vi "Read_raw_inst_setup.vi"(0 "Setup file":path) -> (5 "Board type":T4=enum."NB-MIO-16H", 6 "Local ADAM Channels":string[](array[string]), 8 "Setup string":string, 10 "Ch & spans choices":T5(array[cluster]) {"D" format="%.2f"; "Ch No" min=0; "low limit (-10V)" min=-10 max=10 format="%.2f"; "high limit (10V)" min=-10 max=10 format="%.2f"}, 13 "PWA Data":T1, 14 "Number of Analogue instruments":i32=1, 16 "LDA data":enum16{"No LDA data", "Take LDA data"}(ring)=enum."Take LDA data", 17 "LDA set up":T3={"dimensions"=enum."2D", "Arrival spacing"=FALSE, "Transit time"=FALSE}, 19 "Synchronise Analogue channels with LDA":bool)   [LabVIEW 2010]
uses:
  Controls/Inst_type.ctl
  Controls/Board_Types.ctl
  Controls/PWA_Data.ctl
  Controls/Post_Process.ctl
  Controls/Trigger_Mode.ctl
  Controls/Tunnel_Coordinates.ctl
  Globals/Meas_global.vi
  Globals/LDA_meas_global_1.vi
  Globals/LDA_meas_global_2.vi
  Globals/Trav_pos_global.vi
panel:
  in  "Inst type":T2
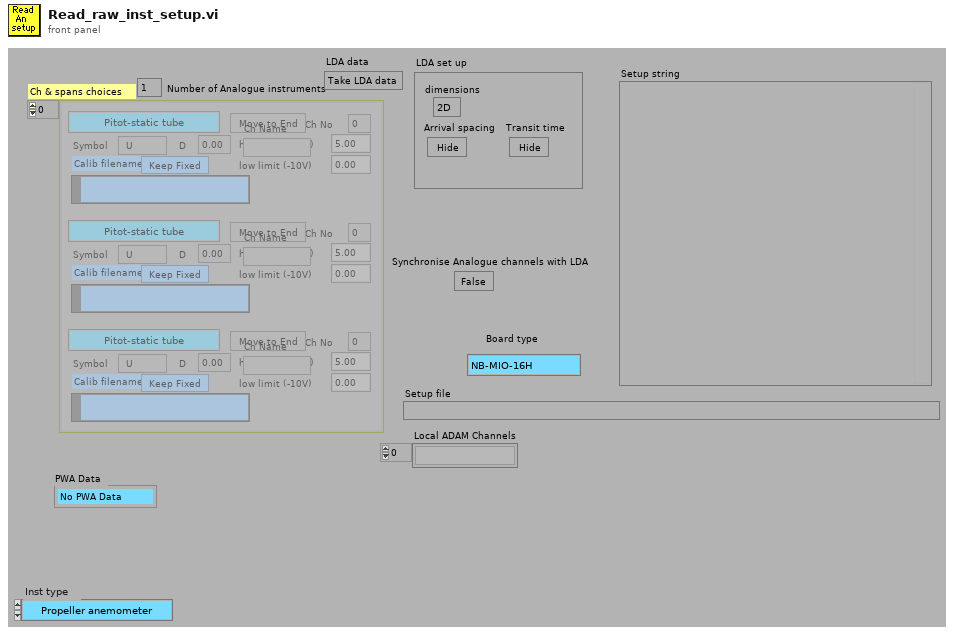
[diagram p1: front panel]
types:
  T1 = typedef "PWA_Data.ctl" = enum16{"No PWA Data", "One Ch PWA"}
  T2 = typedef "Inst_type.ctl" = enum16{"Propeller anemometer", "Raw voltage", "Pressure Transducer", "Pitot-static tube", "Preston tube", "Hot wire", "Cross wire 1", "Cross wire 2", "Generic Linear", "Generic Polynomial", "Generic BackPoly", "Fast FID", "Thermocouple", "Cold wire", "Pulsed Wire", "LDA Vel", "LDA Tran time", "LDA Arr time"}
  T3 = cluster{"dimensions":enum16{"1D", "2D"}, "Arrival spacing":bool, "Transit time":bool}
  T4 = typedef "Board_Types.ctl" = enum16{"Simulate", "NB-MIO-16H", "PCI-MIO-16E", "6000E Series", "USB-92xx", "ADC488", "Lab-NB", "NB-DIO-24", "NI-DAQmx", "Local ADAM", "Server Channels"}
  T5 = cluster{"high limit (10V)":sgl, "low limit (-10V)":sgl, "Ch No":i16, "Calib filename":path, "Inst type":T2, "Symbol":string, "Move channel":bool, "Use Latest":bool, "D":dbl, "Ch Name":string}[]
  T6 = typedef "Post_Process.ctl" = enum16{"Take New Data", "Post Process Raw Data File"}
  T7 = typedef "Trigger_Mode.ctl" = enum16{"Free Running", "Start on Trigger", "Trigger Every Block", "Trigger Every Sample"}
  T8 = typedef "Tunnel_Coordinates.ctl" = enum16{"Work in Tunnel Coordinates", "Work in Model Coordinates"}
  T9 = cluster{"high limit (10V)":sgl, "low limit (-10V)":sgl, "Ch No":i16, "Calib filename":path, "Inst type":T2, "Symbol":string, "Move channel":bool, "Use Latest":bool, "D":dbl, "Ch Name":string}
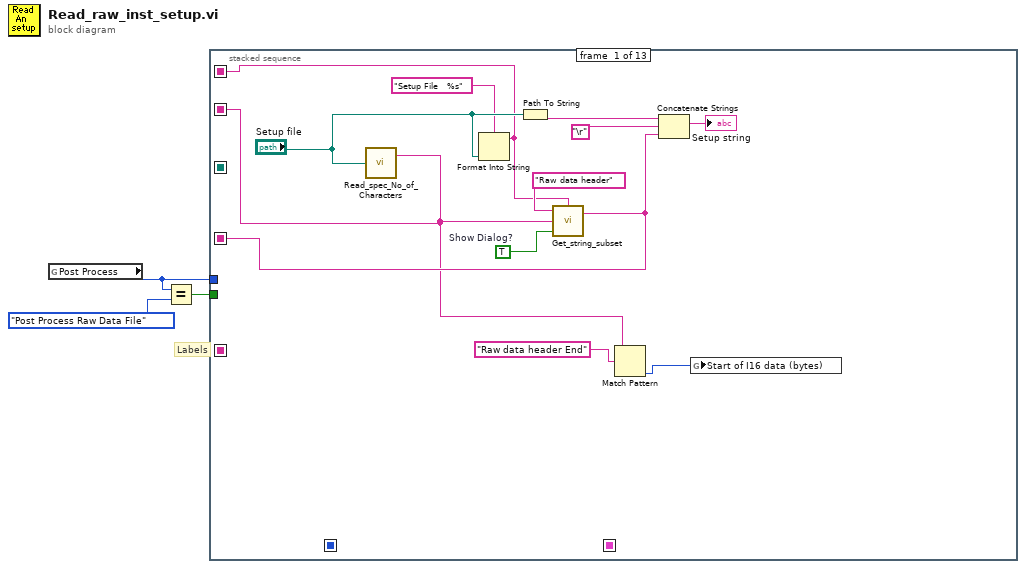
[diagram p0: block diagram]
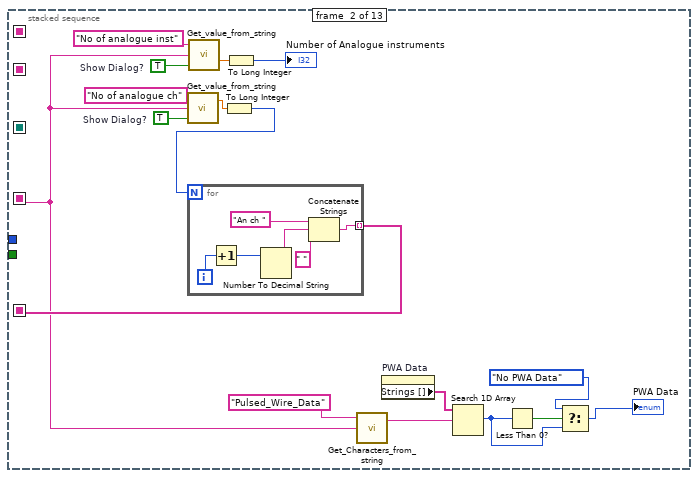
[diagram p2: hidden frame]
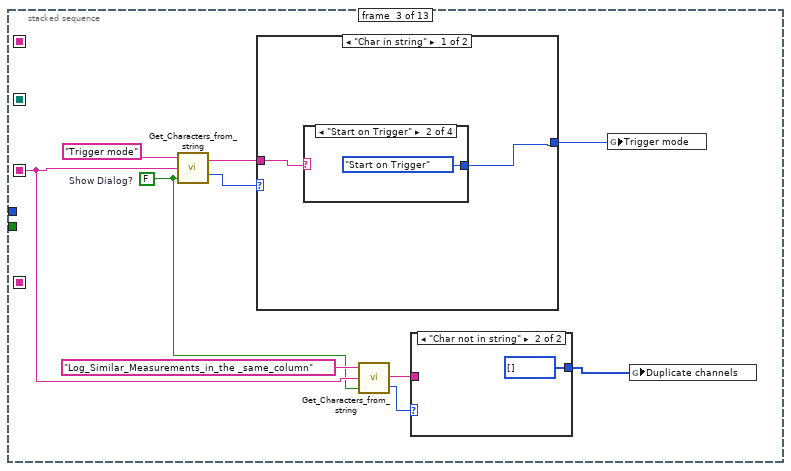
[diagram p3: hidden frame]
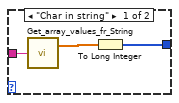
[diagram p4: hidden frame]
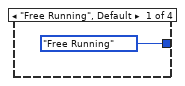
[diagram p5: hidden frame]
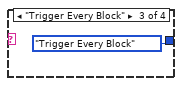
[diagram p6: hidden frame]
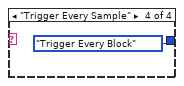
[diagram p7: hidden frame]
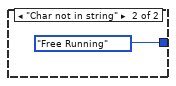
[diagram p8: hidden frame]
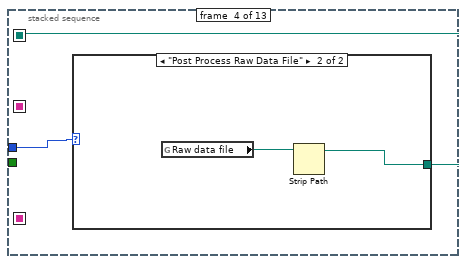
[diagram p9: hidden frame]
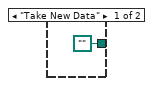
[diagram p10: hidden frame]
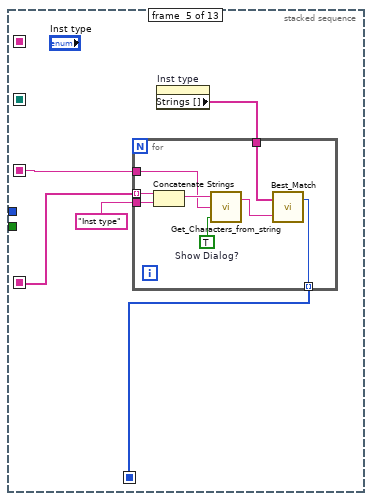
[diagram p11: hidden frame]
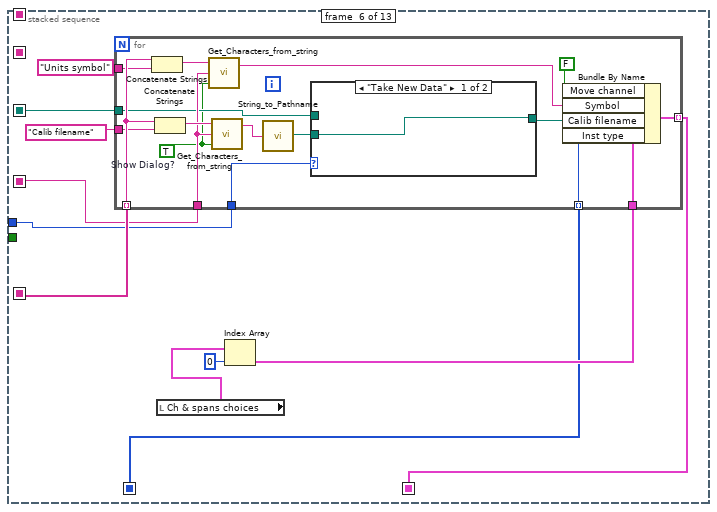
[diagram p12: hidden frame]
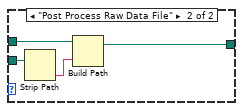
[diagram p13: hidden frame]
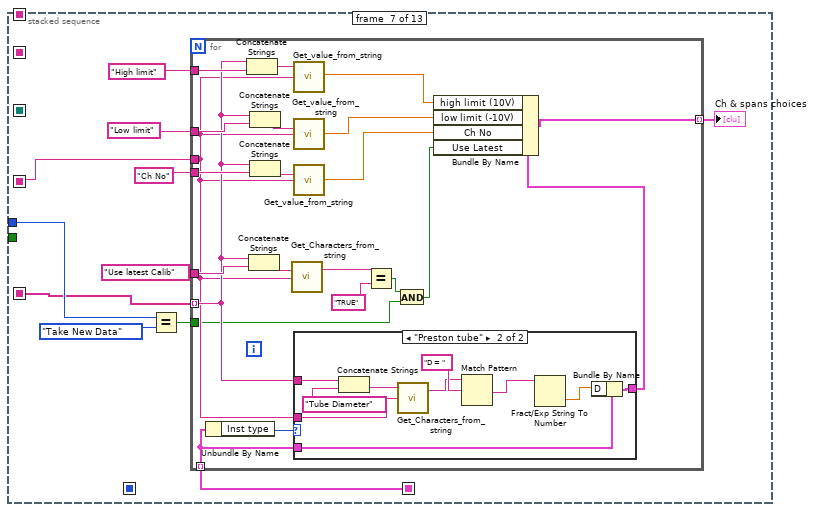
[diagram p14: hidden frame]
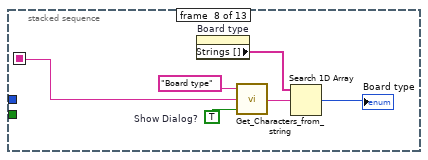
[diagram p16: hidden frame]
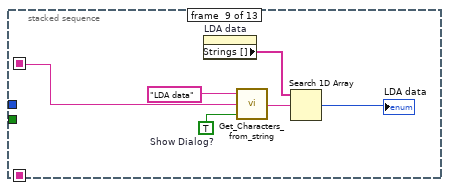
[diagram p17: hidden frame]
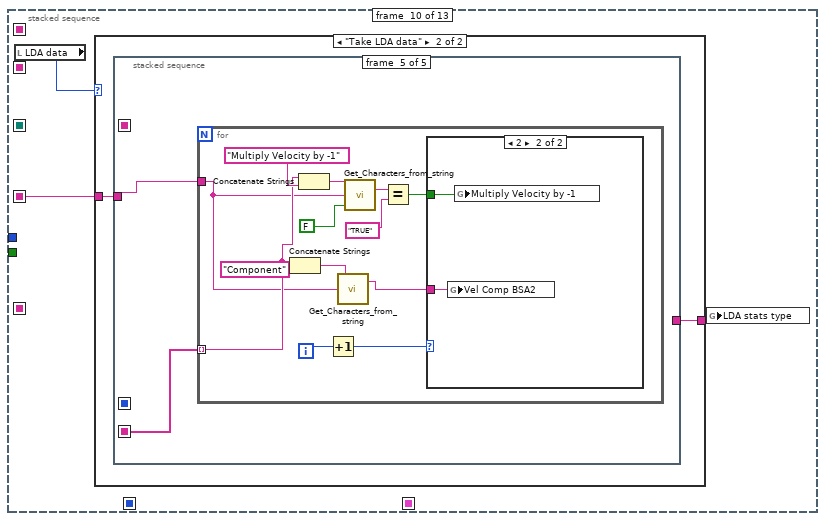
[diagram p18: hidden frame]
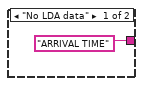
[diagram p19: hidden frame]
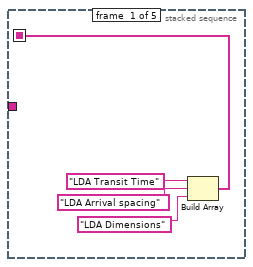
[diagram p20: hidden frame]
diagram:
  # "Labels"
  n1 = global read "Meas_global.vi" "Post Process"() -> (w1:T6)
  n2 = Equal?(x=w1, y=Post_Process."Post Process Raw Data File" ("Post Process")) -> (x = y?=w3:bool)
  n3 = stacked-sequence {
    seq-local: [w13 _ _ _ _ _ _ _ _ _ _ _ _] -> [_ w23 w43 _ w69 w79 w121 w159 w165 w169 w251 w278 w291]
    seq-local: [_ w30 _ _ _ _ _ _ _ _ _ _ _] -> [_ _ _ _ w68 w88 w112 _ _ _ _ _ _]
    seq-local: [_ _ _ _ w65 _ _ _ _ _ _ _ _] -> [_ _ _ _ _ w82 _ _ _ _ _ _ _]
    seq-local: [_ _ _ _ _ w81 _ _ _ _ _ _ _] -> [_ _ _ _ _ _ w120 _ _ _ _ _ _]
    seq-local: [_ _ _ w61 _ _ _ _ _ _ _ _ _] -> [_ _ _ _ _ w80 _ _ _ _ _ _ _]
    seq-local: [w8 _ _ _ _ _ _ _ _ _ _ _ _] -> [_ _ _ _ _ _ _ _ _ _ _ _ w290]
    seq-local: [w4 _ _ _ _ _ _ _ _ _ _ _ _] -> [_ _ _ _ _ _ _ _ _ _ _ w274 _]
    tunnel: w3 -> [_ _ _ _ _ _ _ _ _ _ _ _ w292]
    tunnel: w1 -> [_ _ _ w60 _ w78 w113 _ _ _ _ w275 _]
    frame #0 {
      w10 = TRUE  # Show Dialog?
      n4 = call "Read_spec_No_of_Characters.vi"("Filename"="Setup file") -> ("character string"=w8:string)  [unwired: 1 out]
      n5 = Format Into String(format string="Setup File   %s", "Setup file") -> (resulting string=w4:string)  [unwired: 2 in, 1 out]
      n6 = Path To String(path="Setup file") -> (string=w11:string)
      n7 = call "Get_string_subset.vi"("String Name"=w4, "Show Dialog?"=w10, "String to split"=w8, "File Label"="Raw data header") -> ("Output string"=w13:string)  [unwired: 1 out]
      n8 = Match Pattern(string=w8, regular expression="Raw data header End") -> (offset past match=w7:i32)  [unwired: 4 out]
      n9 = Concatenate Strings(w11, "\r", w13) -> (→"Setup string":string)
      n10 = global write "Meas_global.vi" "Start of I16 data (bytes)"(w7) -> ()
    }
    frame #1 {
      w24 = TRUE  # Show Dialog?
      w25 = TRUE  # Show Dialog?
      n11 = call "Get_value_from_string.vi"("Show Dialog?"=w25, "Input string"=w23, "Variable name"="No of analogue ch") -> ("Value"=w31:dbl)  [unwired: 1 out]
      n12 = call "Get_value_from_string.vi"("Show Dialog?"=w24, "Input string"=w23, "Variable name"="No of analogue inst") -> ("Value"=w28:dbl)  [unwired: 1 out]
      n13 = To Long Integer(number=w31) -> (32bit integer=w26:i32)
      n14 = for {
        N: w26 -> [_]
        tunnel: [w34] -> w30 mode=indexing
        i -> [w36]
        n15 = Increment(x=w36) -> (x+1=w35:i32)
        n16 = Number To Decimal String(number=w35) -> (decimal integer string=w38:string)  [unwired: 1 out]
        n17 = Concatenate Strings("An ch ", w38, " ") -> (w34:string)
      }
      n18 = To Long Integer(number=w28) -> (32bit integer=→"Number of Analogue instruments":i32)
      n19 = call "Get_Characters_from_string.vi"("Input string"=w23, "Variable name"="Pulsed_Wire_Data") -> ("Value"=w20:string)  [unwired: 1 in, 1 out]
      n20 = property on="PWA Data" class="Enum (strict)"() -> ("Strings []"=w21:string[])  [unwired: 2 in, 2 out]
      n21 = Search 1D Array(1D array=w21, element=w20) -> (index of element=w17:i32)  [unwired: 1 out]
      n22 = Less Than 0?(x=w17) -> (x < 0?=w19:bool)
      n23 = Select(t=PWA_Data."No PWA Data" ("PWA Data"), s=w19, f=w17) -> (s? t:f=→"PWA Data":i32)
    }
    frame #2 {
      w42 = FALSE  # Show Dialog?
      n24 = call "Get_Characters_from_string.vi"("Show Dialog?"=w42, "Input string"=w43, "Variable name"="Trigger mode") -> ("Status"=w47:enum16{"Char in string", "Char not in string"}, "Value"=w46:string)
      n25 = case shown="\"Char in string\"" w47 {
        tunnel: [w53 Trigger_Mode."Free Running" ("Trigger mode")] -> w45
        tunnel: w46 -> [w54 _]
        frame "Char in string" {
          n26 = case shown="\"Start on Trigger\"" w54 {
            tunnel: [Trigger_Mode."Free Running" ("Trigger mode") Trigger_Mode."Start on Trigger" ("Trigger mode") Trigger_Mode."Trigger Every Block" ("Trigger mode") Trigger_Mode."Trigger Every Block" ("Trigger mode")] -> w53
            frame "Free Running", Default {
            }
            frame "Start on Trigger" {
            }
            frame "Trigger Every Block" {
            }
            frame "Trigger Every Sample" {
            }
          }
        }
        frame "Char not in string" {
        }
      }
      n27 = call "Get_Characters_from_string.vi"("Show Dialog?"=w42, "Input string"=w43, "Variable name"="Log_Similar_Measurements_in_the _same_column") -> ("Status"=w39:enum16{"Char in string", "Char not in string"}, "Value"=w41:string)
      n28 = case shown="\"Char not in string\"" w39 {
        tunnel: w41 -> [w51 _]
        tunnel: [w49 i32[] []] -> w40
        frame "Char in string" {
          n29 = call "Get_array_values_fr_String.vi"("String Value"=w51) -> ("Numeric Array"=w50:dbl[])  [unwired: 1 out]
          n30 = To Long Integer(number=w50) -> (32bit integer=w49:i32[])
        }
        frame "Char not in string" {
        }
      }
      n31 = global write "Meas_global.vi" "Trigger mode"(w45) -> ()
      n32 = global write "Meas_global.vi" "Duplicate channels"(w40) -> ()
    }
    frame #3 {
      n33 = case shown="\"Post Process Raw Data File\"" w60 {
        tunnel: [path "" ("stripped path") w63] -> w61
        frame "Take New Data" {
        }
        frame "Post Process Raw Data File" {
          n34 = global read "Meas_global.vi" "Raw data file"() -> (w64:path)
          n35 = Strip Path(path=w64) -> (stripped path=w63:path)  [unwired: 1 out]
        }
      }
    }
    frame #4 {
      n36 = property on="Inst type" class="Enum (strict)"() -> ("Strings []"=w66:string[])  [unwired: 2 in, 2 out]
      n37 = for {
        tunnel: w69 -> [w76]
        tunnel: w66 -> [w72]
        tunnel: w68 -> [w75] mode=indexing
        tunnel: "Inst type" -> [w74]
        tunnel: [w70] -> w65 mode=indexing
        w73 = TRUE  # Show Dialog?
        n38 = Concatenate Strings(w75, w74) -> (w77:string)
        n39 = call "Get_Characters_from_string.vi"("Show Dialog?"=w73, "Input string"=w76, "Variable name"=w77) -> ("Value"=w71:string)  [unwired: 1 out]
        n40 = call "Best_Match.vi"("Input String"=w71, "String Options"=w72) -> ("index of element"=w70:i32)  [unwired: 1 out]
      }
    }
    frame #5 {
      n41 = local read "Ch & spans choices"() -> (w84:T5)
      n42 = Index Array(array=w84, index=0) -> (element=w83:T9)
      n43 = for {
        tunnel: w88 -> [w103] mode=indexing
        tunnel: "Calib filename" -> [w102]
        tunnel: "Units symbol" -> [w101]
        tunnel: w83 -> [w100]
        tunnel: w82 -> [w98] mode=indexing
        tunnel: [w97] -> w81 mode=indexing
        tunnel: w79 -> [w96]
        tunnel: w78 -> [w95]
        tunnel: w80 -> [w94]
        w91 = TRUE  # Show Dialog?
        n44 = Concatenate Strings(w103, w101) -> (w105:string)
        n45 = Concatenate Strings(w103, w102) -> (w104:string)
        n46 = call "Get_Characters_from_string.vi"("Show Dialog?"=w91, "Input string"=w96, "Variable name"=w105) -> ("Value"=w99:string)  [unwired: 1 out]
        n47 = call "Get_Characters_from_string.vi"("Show Dialog?"=w91, "Input string"=w96, "Variable name"=w104) -> ("Value"=w90:string)  [unwired: 1 out]
        n48 = call "String_to_Pathname.vi"("Input String"=w90) -> ("path"=w89:path)
        n49 = case shown="\"Take New Data\"" w95 {
          tunnel: w89 -> [w106 w110]
          tunnel: w94 -> [_ w107]
          tunnel: [w106 w108] -> w93
          frame "Take New Data" {
          }
          frame "Post Process Raw Data File" {
            n50 = Strip Path(path=w110) -> (name=w109:string)  [unwired: 1 out]
            n51 = Build Path(base path=w107, name or relative path=w109) -> (appended path=w108:path)
          }
        }
        n52 = Bundle By Name(cluster=w100, "Move channel"=FALSE, "Symbol"=w99, "Calib filename"=w93, "Inst type"=w98) -> (w97:T9)
      }
    }
    frame #6 {
      n53 = Equal?(x=w113, y=Post_Process."Take New Data" ("Post Process")) -> (x = y?=w111:bool)
      n54 = for {
        tunnel: "Low limit" -> [w143]
        tunnel: "High limit" -> [w142]
        tunnel: w120 -> [w124] mode=indexing
        tunnel: [w134] -> w119 mode=indexing
        tunnel: w121 -> [w126]
        tunnel: "Ch No" -> [w138]
        tunnel: "Use latest Calib" -> [w132]
        tunnel: w112 -> [w127] mode=indexing
        tunnel: w111 -> [w125]
        n55 = Unbundle By Name(w124) -> ("Inst type"=w128:T2)
        n56 = Concatenate Strings(w127, w142) -> (w141:string)
        n57 = Concatenate Strings(w127, w132) -> (w133:string)
        n58 = Concatenate Strings(w127, w143) -> (w140:string)
        n59 = Concatenate Strings(w127, w138) -> (w139:string)
        n60 = call "Get_Characters_from_string.vi"("Input string"=w126, "Variable name"=w133) -> ("Value"=w131:string)  [unwired: 1 in, 1 out]
        n61 = call "Get_value_from_string.vi"("Input string"=w126, "Variable name"=w141) -> ("Value"=w137:dbl)  [unwired: 1 in, 1 out]
        n62 = call "Get_value_from_string.vi"("Input string"=w126, "Variable name"=w140) -> ("Value"=w136:dbl)  [unwired: 1 in, 1 out]
        n63 = call "Get_value_from_string.vi"("Input string"=w126, "Variable name"=w139) -> ("Value"=w135:dbl)  [unwired: 1 in, 1 out]
        n64 = case shown="\"Preston tube\"" w128 {
          tunnel: w127 -> [_ w154]
          tunnel: w126 -> [_ w149]
          tunnel: w124 -> [w144 w152]
          tunnel: [w144 w151] -> w123
          frame "Propeller anemometer", Default {
          }
          frame "Preston tube" {
            n65 = Concatenate Strings(w154, "Tube Diameter") -> (w150:string)
            n66 = call "Get_Characters_from_string.vi"("Input string"=w149, "Variable name"=w150) -> ("Value"=w147:string)  [unwired: 1 in, 1 out]
            n67 = Match Pattern(string=w147, regular expression="D = " ("String to match")) -> (after substring=w146:string)  [unwired: 4 out]
            n68 = Fract/Exp String To Number(string=w146) -> (number=w145:dbl)  [unwired: 4 out]
            n69 = Bundle By Name(cluster=w152, "D"=w145) -> (w151:T9)
          }
        }
        n70 = Equal?(x=w131, y="TRUE") -> (x = y?=w129:bool)
        n71 = And(x=w129, y=w125) -> (x .and. y?=w122:bool)
        n72 = Bundle By Name(cluster=w123, "high limit (10V)"=w137, "low limit (-10V)"=w136, "Ch No"=w135, "Use Latest"=w122) -> (w134:T9)
      }
      "Ch & spans choices" <- w119
    }
    frame #7 {
      w156 = TRUE  # Show Dialog?
      n73 = property on="Board type" class="Enum (strict)"() -> ("Strings []"=w155:string[])  [unwired: 2 in, 2 out]
      n74 = call "Get_Characters_from_string.vi"("Show Dialog?"=w156, "Input string"=w159, "Variable name"="Board type") -> ("Value"=w160:string)  [unwired: 1 out]
      n75 = Search 1D Array(1D array=w155, element=w160) -> (index of element=→"Board type":i32)  [unwired: 1 out]
    }
    frame #8 {
      w162 = TRUE  # Show Dialog?
      n76 = property on="LDA data" class="Enum (strict)"() -> ("Strings []"=w161:string[])  [unwired: 2 in, 2 out]
      n77 = call "Get_Characters_from_string.vi"("Show Dialog?"=w162, "Input string"=w165, "Variable name"="LDA data" ("Label for characters")) -> ("Value"=w166:string)  [unwired: 1 out]
      n78 = Search 1D Array(1D array=w161, element=w166) -> (index of element=→"LDA data":i32)  [unwired: 1 out]
    }
    frame #9 {
      n79 = local read "LDA data"() -> (w168:enum16{"No LDA data", "Take LDA data"})
      n80 = case shown="\"Take LDA data\"" w168 {
        tunnel: w169 -> [_ w172]
        tunnel: ["ARRIVAL TIME" ("Adam client setup name") w171] -> w167
        frame "No LDA data" {
        }
        frame "Take LDA data" {
          n81 = stacked-sequence {
            seq-local: [_ w178 _ _ _] -> [_ _ _ w222 _]
            seq-local: [_ _ _ w221 _] -> [_ _ _ _ w232]
            seq-local: [w173 _ _ _ _] -> [_ w181 _ _ _]
            tunnel: w172 -> [_ w177 w211 _ w233]
            tunnel: [_ _ w210 _ _] -> w171
            frame #0 {
              n82 = Build Array("LDA Transit Time", "LDA Arrival spacing", "LDA Dimensions") -> (w173:string[])
            }
            frame #1 {
              n83 = local read "LDA set up"() -> (w180:T3)
              n84 = for {
                tunnel: w181 -> [w187] mode=indexing
                shift-right: [w184] -> w179
                shift-left: w180 -> [w185]
                tunnel: w177 -> [w182]
                n85 = call "Get_Characters_from_string.vi"("Input string"=w182, "Variable name"=w187) -> ("Status"=w186:enum16{"Char in string", "Char not in string"}, "Value"=w183:string)  [unwired: 1 in]
                n86 = case shown="\"Char in string\"" w186 {
                  tunnel: w187 -> [w191 _]
                  tunnel: w185 -> [w190 w209]
                  tunnel: [w189 w209] -> w184
                  tunnel: w183 -> [w188 _]
                  frame "Char in string" {
                    n87 = case shown="\"LDA Arrival spacing\"" w191 {
                      tunnel: w190 -> [w195 w198 w203 w208]
                      tunnel: [w194 w198 w202 w207] -> w189
                      tunnel: w188 -> [w193 _ w201 w206]
                      frame "LDA Dimensions" {
                        n88 = case shown="\"2D\", Default" w193 {
                          tunnel: [enum16{"1D", "2D"}."1D" ("Bundle Element") enum16{"1D", "2D"}."2D" ("Bundle Element")] -> w192
                          frame "1D" {
                          }
                          frame "2D", Default {
                          }
                        }
                        n89 = Bundle By Name(cluster=w195, "dimensions"=w192) -> (w194:T3)
                      }
                      frame "No Match", Default {
                      }
                      frame "LDA Arrival spacing" {
                        n90 = Equal?(x=w201, y="TRUE") -> (x = y?=w199:bool)
                        n91 = Bundle By Name(cluster=w203, "Arrival spacing"=w199) -> (w202:T3)
                      }
                      frame "LDA Transit Time" {
                        n92 = Equal?(x=w206, y="TRUE") -> (x = y?=w204:bool)
                        n93 = Bundle By Name(cluster=w208, "Transit time"=w204) -> (w207:T3)
                      }
                    }
                  }
                  frame "Char not in string" {
                  }
                }
              }
              "LDA set up" <- w179
              n94 = Unbundle By Name(w179) -> ("dimensions"=w178:enum16{"1D", "2D"})
            }
            frame #2 {
              n95 = call "Get_Characters_from_string.vi"("Input string"=w211, "Variable name"="LDA stats weighting") -> ("Status"=w214:enum16{"Char in string", "Char not in string"}, "Value"=w213:string)  [unwired: 1 in]
              n96 = case shown="\"Char in string\"" w214 {
                tunnel: "ARRIVAL TIME" ("Adam client setup name") -> [w218 w220]
                tunnel: w213 -> [w217 _]
                tunnel: [w216 w220] -> w210
                frame "Char in string" {
                  n97 = Empty String/Path?(string/path=w217) -> (empty?=w219:bool)
                  n98 = Select(t=w218, s=w219, f=w217) -> (s? t:f=w216:string)
                }
                frame "Char not in string" {
                }
              }
            }
            frame #3 {
              n99 = case shown="\"1D\"" w222 {
                tunnel: [1 2] -> w223
                frame "1D" {
                }
                frame "2D" {
                }
              }
              n100 = for {
                N: w223 -> [_]
                tunnel: [w225] -> w221 mode=indexing
                i -> [w227]
                n101 = Increment(x=w227) -> (x+1=w226:i32)
                n102 = Number To Decimal String(number=w226) -> (decimal integer string=w229:string)  [unwired: 1 out]
                n103 = Concatenate Strings("BSA ", w229, " ") -> (w225:string)
              }
            }
            frame #4 {
              n104 = for {
                tunnel: w233 -> [w235]
                tunnel: w232 -> [w236] mode=indexing
                i -> [w245]
                n105 = Concatenate Strings(w236, "Component") -> (w246:string)
                n106 = Concatenate Strings(w236, "Multiply Velocity by -1") -> (w240:string)
                n107 = Increment(x=w245) -> (x+1=w242:i32)
                n108 = call "Get_Characters_from_string.vi"("Input string"=w235, "Variable name"=w246) -> ("Value"=w243:string)  [unwired: 1 in, 1 out]
                n109 = call "Get_Characters_from_string.vi"("Show Dialog?"=FALSE, "Input string"=w235, "Variable name"=w240) -> ("Value"=w238:string)  [unwired: 1 out]
                n110 = Equal?(x=w238, y="TRUE") -> (x = y?=w234:bool)
                n111 = case shown="2" w242 {
                  tunnel: w243 -> [w248 w250]
                  tunnel: w234 -> [w247 w249]
                  frame 1, Default {
                    n112 = global write "LDA_meas_global_1.vi" "Vel Comp BSA1"(w248) -> ()
                    n113 = global write "LDA_meas_global_1.vi" "Multiply Velocity by -1"(w247) -> ()
                  }
                  frame 2 {
                    n114 = global write "LDA_meas_global_2.vi" "Vel Comp BSA2"(w250) -> ()
                    n115 = global write "LDA_meas_global_2.vi" "Multiply Velocity by -1"(w249) -> ()
                  }
                }
              }
            }
          }
        }
      }
      n116 = global write "LDA_meas_global_1.vi" "LDA stats type"(w167) -> ()
    }
    frame #10 {
      n117 = Build Array("Synchronise with LDA") -> (w261:string[])
      n118 = Build Array("FALSE", "TRUE") -> (w258:string[])
      n119 = call "Get_value_from_string.vi"("Input string"=w251, "Variable name"="Sync Delay Time (ms)" ("Label for characters")) -> ("Status"=w253:enum16{"Char in string", "Char not in string"}, "Value"=w252:dbl)  [unwired: 1 in]
      n120 = case shown="\"Char in string\"" w253 {
        tunnel: w252 -> [w263 _]
        frame "Char in string" {
          n121 = global write "LDA_meas_global_1.vi" "Sync Delay Time (ms)"(w263) -> ()
        }
        frame "Char not in string" {
        }
      }
      n122 = Build Array(FALSE, TRUE) -> (w255:bool[])
      n123 = for {
        tunnel: w251 -> [w271]
        tunnel: w261 -> [w267] mode=indexing
        tunnel: w258 -> [w266]
        tunnel: w255 -> [w265]
        i -> [w269]
        w264 = TRUE  # Show Dialog?
        n124 = call "Get_Characters_from_string.vi"("Show Dialog?"=w264, "Input string"=w271, "Variable name"=w267) -> ("Value"=w272:string)  [unwired: 1 out]
        n125 = Search 1D Array(1D array=w266, element=w272) -> (index of element=w270:i32)  [unwired: 1 out]
        n126 = Index Array(array=w265, index=w270) -> (element=w268:bool)
        n127 = case shown="1" w269 {
          tunnel: w268 -> [w273 _]
          frame 0, Default {
            "Synchronise Analogue channels with LDA" <- w273
          }
          frame 1 {
          }
        }
      }
    }
    frame #11 {
      n128 = Build Array("Local ADAM Channels") -> (w277:string[])
      n129 = for {
        tunnel: w278 -> [w284]
        tunnel: w277 -> [w283] mode=indexing
        tunnel: w275 -> [w280]
        tunnel: w274 -> [w279]
        i -> [w282]
        n130 = call "Get_string_subset.vi"("String Name"=w279, "String to split"=w284, "File Label"=w283) -> ("Output string"=w288:string)  [unwired: 1 in, 1 out]
        n131 = Initialize Array("") -> (w281:string[])  [unwired: 1 out]
        n132 = Spreadsheet String To Array(format string="%s", spreadsheet string=w288, array type (2D Dbl)=w281) -> (array=w285:string[])  [unwired: 1 out]
        n133 = case shown="0, Default" w282 {
          tunnel: w285 -> [w289]
          tunnel: w280 -> [_]
          frame 0, Default {
            "Local ADAM Channels" <- w289
          }
        }
      }
    }
    frame #12 {
      n134 = case shown="True" w292 {
        tunnel: w291 -> [_ w298]
        tunnel: w290 -> [_ w293]
        frame False {
        }
        frame True {
          w297 = FALSE  # Show Dialog?
          n135 = call "Get_Characters_from_string.vi"("Show Dialog?"=w297, "Input string"=w298, "Variable name"="Coordinate_System" ("Label for characters")) -> ("Status"=w296:enum16{"Char in string", "Char not in string"}, "Value"=w295:string)
          n136 = case shown="\"Char not in string\"" w296 {
            tunnel: w295 -> [w301 _]
            tunnel: [w300 w304] -> w294
            tunnel: w293 -> [_ w306]
            frame "Char in string" {
              n137 = case shown="\"Work in Model Coordinates\"" w301 {
                tunnel: [Tunnel_Coordinates."Work in Model Coordinates" ("Work in Tunnel Coordinates?") Tunnel_Coordinates."Work in Tunnel Coordinates" ("Work in Tunnel Coordinates?")] -> w300
                frame "Work in Model Coordinates" {
                }
                frame "Work in Tunnel Coordinates", Default {
                }
              }
            }
            frame "Char not in string" {
              n138 = Concatenate Strings("X Pos (Model)", "\t", "Y Pos (Model)") -> (w307:string)
              n139 = Match Pattern(string=w306, regular expression=w307) -> (offset past match=w305:i32)  [unwired: 4 out]
              n140 = case shown="-1" w305 {
                tunnel: [Tunnel_Coordinates."Work in Model Coordinates" ("Work in Tunnel Coordinates?") Tunnel_Coordinates."Work in Tunnel Coordinates" ("Work in Tunnel Coordinates?")] -> w304
                frame 0, Default {
                }
                frame -1 {
                }
              }
            }
          }
          n141 = global write "Trav_pos_global.vi" "Work in Tunnel Coordinates?"(w294) -> ()
        }
      }
    }
  }
